vi "UI_init.vi"() -> ()   [LabVIEW 2018]
uses:
  UI Data.ctl
panel:
  out "error out":cluster{"状态":bool, "代码":i32, "源":string}
  in  "UI引用":T1
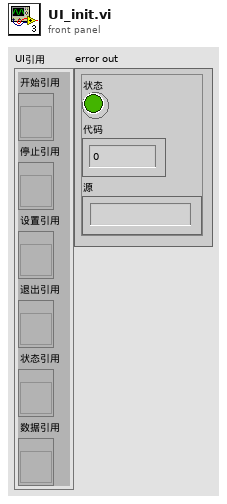
[diagram p1: front panel]
types:
  T1 = typedef "UI Data.ctl" = cluster{"开始引用":refnum<vi>, "停止引用":refnum<vi>, "设置引用":refnum<vi>, "退出引用":refnum<vi>, "状态引用":refnum<vi>, "数据引用":refnum<vi>}
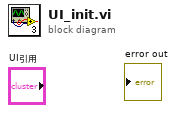
[diagram p0: block diagram]
diagram:
